vi "Build Time Filter.vi"(8 "error in (no error)":errorcluster, 9 "Comparison Timestamp":timestamp, 10 "Comparison Method":enum16{"Before", "After"}(ring), 11 "Time Filters in":refnum<class "Time Filters.lvclass">) -> (0 "error out":errorcluster, 3 "Time Filters out":refnum<class "Time Filters.lvclass">)   [LabVIEW 2016, in "Assert API Components.lvlib" / "Time Filters.lvclass"]
uses:
  Time Filters.lvclass
  Time Filters.lvclass/Time Filters.ctl
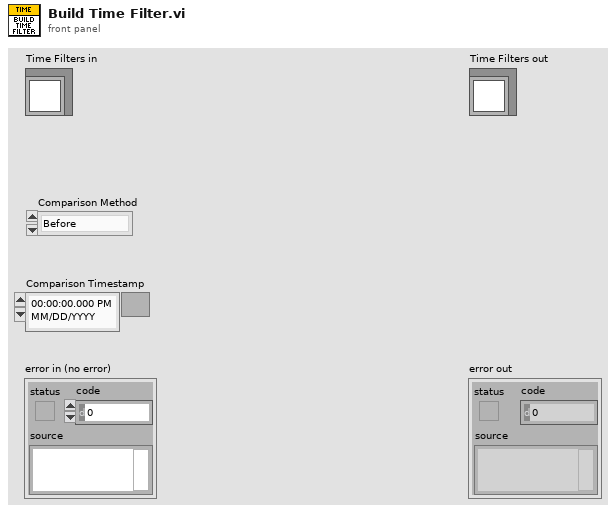
[diagram p1: front panel]
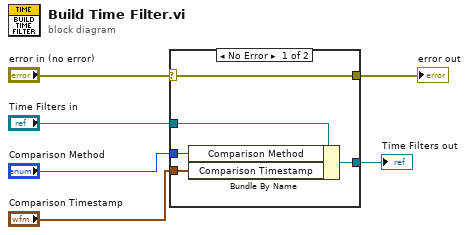
[diagram p0: block diagram]
diagram:
  n1 = case shown="No Error" "error in (no error)" {
    selector: "error in (no error)" -> [w10 w13]
    tunnel: [w10 w13] -> w5
    tunnel: [w9 w12] -> w3
    tunnel: "Time Filters in" -> [w11 w12]
    tunnel: "Comparison Method" -> [w8 _]
    tunnel: "Comparison Timestamp" -> [w7 _]
    frame No Error {
      n2 = Bundle By Name(cluster=w11, "Comparison Method"=w8, "Comparison Timestamp"=w7) -> (w9:refnum<class "Time Filters.lvclass">)
    }
    frame Error {
    }
  }
  "error out" <- w5
  "Time Filters out" <- w3
